vi "persistence front panel.vi"() -> ()   [LabVIEW 2025]
doc: "Author: Scott Hannahs <sth@magnet.fsu.edu>\n\nThis software is licensed for use under the “MIT License\"\nCopyright (c) 2025 Scott Hannahs, sth@sth@magnet.sthnet.net\n\nPermission is hereby granted, free of charge, to any person obtaining a copy of this software and associated documentation files (the \"Software\"), to deal in the Software without restriction, including without limitation the rights to use, copy, modify, merge, publish, distribute, sublicense, and/or sell copies of the Software, and to permit persons to whom the Software is furnished to do so, subject to the following conditions: The above copyright notice and this permission notice shall be included in all copies or substantial portions of the Software.\n\nTHE SOFTWARE IS PROVIDED \"AS IS\", WITHOUT WARRANTY OF ANY KIND, EXPRESS OR IMPLIED, INCLUDING BUT NOT LIMITED TO THE WARRANTIES OF MERCHANTABILITY, FITNESS FOR A PARTICULAR PURPOSE AND NONINFRINGEMENT. IN NO EVENT SHALL THE AUTHORS OR COPYRIGHT HOLDERS BE LIABLE FOR ANY CLAIM, DAMAGES OR OTHER LIABILITY, WHETHER IN AN ACTION OF CONTRACT, TORT OR OTHERWISE, ARISING FROM, OUT OF OR IN CONNECTION WITH THE SOFTWARE OR THE USE OR OTHER DEALINGS IN THE SOFTWARE."
panel:
  out "Persistence Status":string
  out "Persistent":bool
  in  "Return from persistence":bool
  in  "Make Persistent":bool
  out "Switch Heater\nError":bool
  out "Switch heater \nconfirmed":bool
  out "Switch Heater":bool
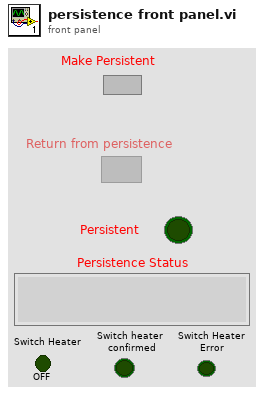
[diagram p1: front panel]
types:
  T1 = enum16{"Always On", "Always Off", "Off While Running"}
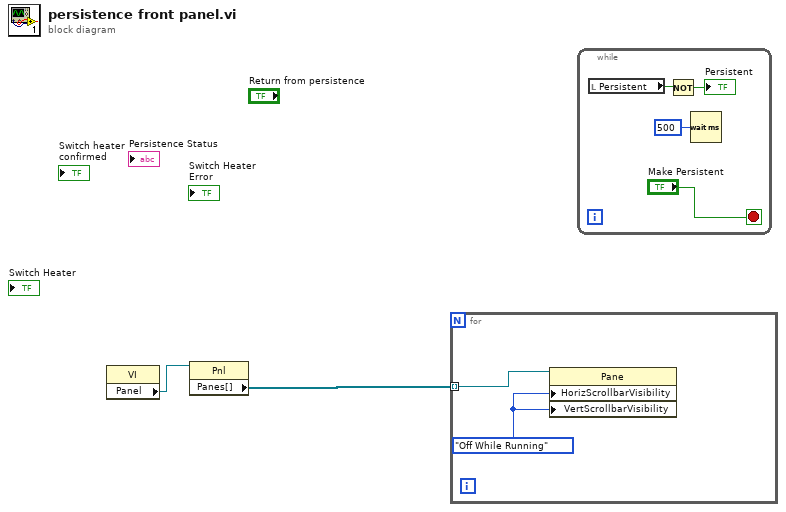
[diagram p0: block diagram]
diagram:
  n1 = property class="VI"() -> ("Panel"=w2:refnum<vi>)  [unwired: 2 in, 2 out]
  n2 = property class="Pnl"(reference=w2) -> ("Panes[]"=w1:refnum<vi>[])  [unwired: 1 in, 2 out]
  n3 = for {
    tunnel: w1 -> [w4] mode=indexing
    w3 = T1."Off While Running" ("Vertical Scrollbar Visibility")
    n4 = property class="Pane"(reference=w4, "HorizScrollbarVisibility"=w3, "VertScrollbarVisibility"=w3) -> ()  [unwired: 1 in, 2 out]
  }
  n5 = while {
    stop <- "Make Persistent" stop-if-true
    n6 = local read "Persistent"() -> (w5:bool)
    n7 = Not(x=w5) -> (.not. x?=→"Persistent":bool)
    n8 = Wait (ms)(milliseconds to wait=u32 500) -> ()  [unwired: 1 out]
  }
